vi "pruebas.vi"() -> ()   [LabVIEW 2025]
panel:
  out "concatenated string":string
  in  "Pin":i16
  out "read buffer":string
  in  "stop":bool
  out "return count":u16
  in  "Boolean":bool
  out "error out":errorcluster
  out "VISA resource name out":refnum<visa-resource-name>
  out "find list":string[](array[string])
  in  "error in (no error)":errorcluster
  in  "Selector":string(combo)
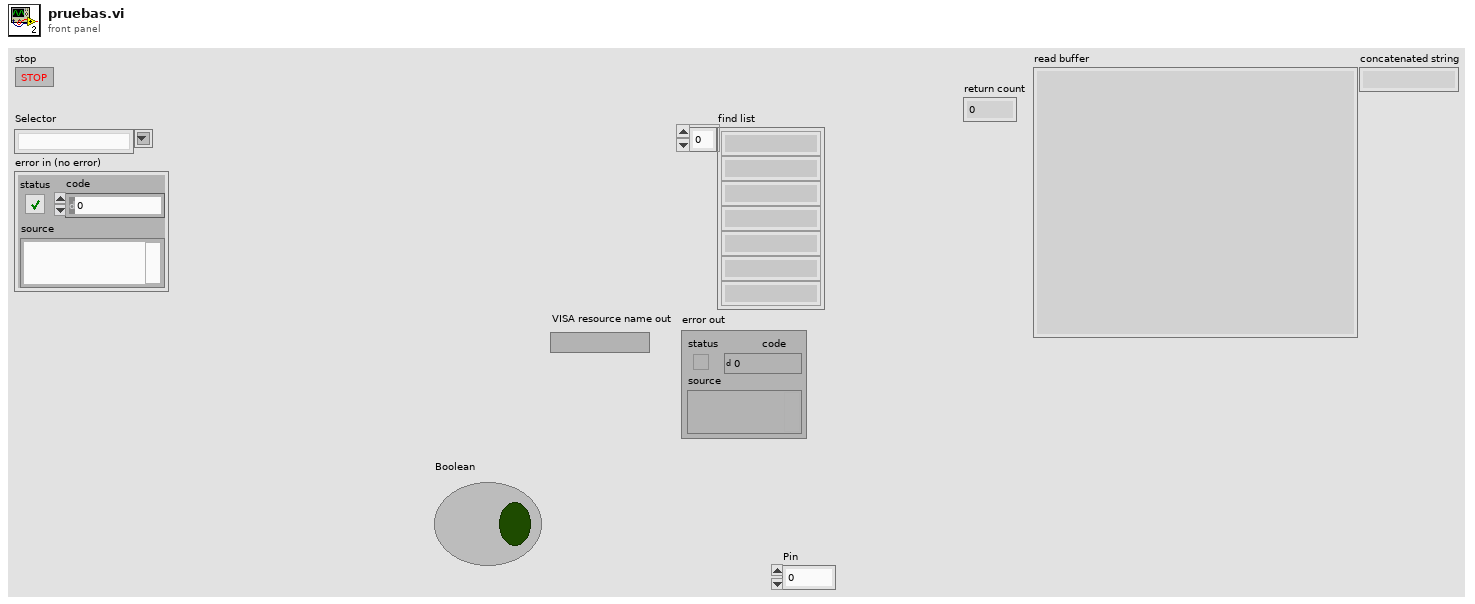
[diagram p1: front panel]
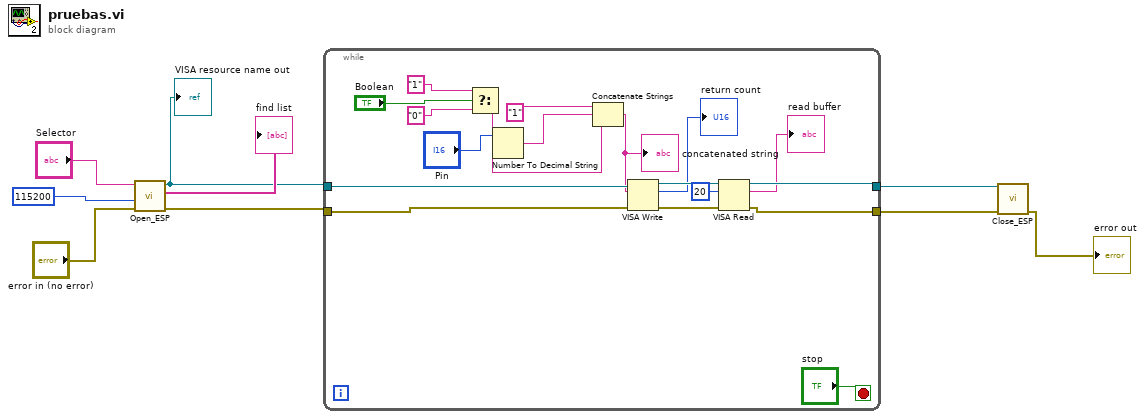
[diagram p0: block diagram]
diagram:
  n1 = call "Open_ESP.vi"("error in (no error)"="error in (no error)", "Baudrate"=i64 115200, "Selector"="Selector") -> ("error out"=w5:errorcluster, "find list"=→"find list":string[], "VISA resource name out"=w6:refnum<visa-resource-name>)  [unwired: 6 in]
  "VISA resource name out" <- w6
  n2 = while {
    tunnel: w6 -> [w27]
    tunnel: [w22] -> w3
    tunnel: w5 -> [w26]
    tunnel: [w21] -> w2
    stop <- "stop" stop-if-true
    n3 = Select(t="1", s="Boolean", f="0") -> (s? t:f=w11:string)
    n4 = Number To Decimal String(number="Pin") -> (decimal integer string=w14:string)  [unwired: 1 in]
    n5 = Concatenate Strings("1", w14, w11) -> (w10:string)
    "concatenated string" <- w10
    n6 = VISA Write(VISA resource name=w27, write buffer=w10, error in (no error)=w26) -> (VISA resource name out=w23:refnum<visa-resource-name>, return count=→"return count":u32, error out=w20:errorcluster)
    n7 = VISA Read(VISA resource name=w23, byte count=u32 20, error in (no error)=w20) -> (VISA resource name out=w22:refnum<visa-resource-name>, read buffer=→"read buffer":string, error out=w21:errorcluster)  [unwired: 1 out]
  }
  n8 = call "Close_ESP.vi"("error in (no error)"=w2, "VISA resource name"=w3) -> ("error out"=→"error out":errorcluster)  [unwired: 9 in]
